vi "wrapper.vi"(8 "error in (no error)":errorcluster, 10 "Actor in":refnum<class "Actor.lvclass">, 11 "Change Frequency MSG in":refnum<class "Change Frequency MSG.lvclass">) -> (0 "error out":errorcluster, 3 "Actor out":refnum<class "Actor.lvclass">)   [LabVIEW 2014, in "Calibration.lvlib" / "Change Frequency MSG.lvclass"]
uses:
  Change Frequency MSG.lvclass
  <vilib>/ActorFramework/Actor/Actor.lvclass
  O3 Frequency Train Actor.lvclass
  SuperActor/SuperActor.lvclass/SuperActor.ctl
  O3 Frequency Train Actor.lvclass/O3 Frequency Train Actor.ctl
  Change Frequency MSG.lvclass/Change Frequency MSG.ctl
  SuperActor/Read CVT Session.vi
  SuperActor/Read Log Session.vi
  Accessors/Read FreqNotifier.vi
  <userlib>/_Session Fwk/Session - Root.lvclass
  reusable/Session APIs/Session Log/System Log.lvclass
  reusable/Session APIs/CVT/CVT.lvclass
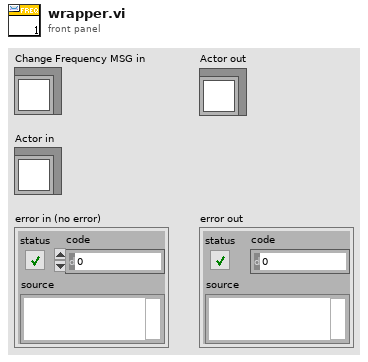
[diagram p1: front panel]
types:
  T1 = typedef "Session - Root.lvclass/Session Handle.ctl" = refnum<data-value>
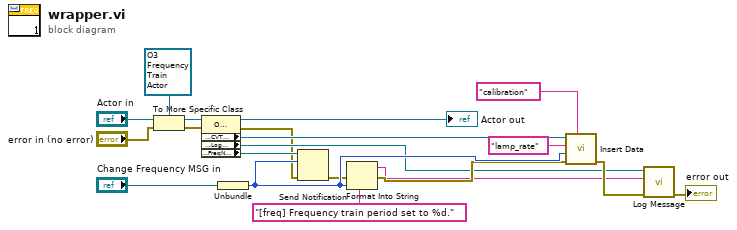
[diagram p0: block diagram]
diagram:
  n1 = To More Specific Class(target class=refnum<class "O3 Frequency Train Actor.lvclass"> refnum ("Calibration.lvlib:O3 Frequency Train Actors"), reference="Actor in", error in="error in (no error)") -> (specific class reference=w4:refnum<class "O3 Frequency Train Actor.lvclass">, error out=w5:errorcluster)
  n2 = property class="O3 Frequency Train Actors"(reference=w4, error in=w5) -> (reference out=→"Actor out":refnum<class "O3 Frequency Train Actor.lvclass">, error out=w7:errorcluster, "Accessors:CVT Session"=w15:T1, "Accessors:Log Session"=w14:T1, "Accessors:FreqNotifier"=w11:refnum<notifier>)
  n3 = Unbundle("Change Frequency MSG in") -> (w20:i64)
  n4 = Send Notification(notification=w20, notifier=w11, error in (no error)=w7) -> (error out=w13:errorcluster)  [unwired: 1 out]
  n5 = Format Into String(format string="[freq] Frequency train period set to %d.", error in=w13, w20) -> (resulting string=w9:string, error out=w16:errorcluster)  [unwired: 1 in]
  n6 = call "Insert Data.vi"("Group"="calibration", "error in"=w16, "Data"=w20, "tag"="lamp_rate", "CVT Session In"=w15) -> ("error out"=w17:errorcluster)  [unwired: 5 in, 1 out]
  n7 = call "Log Message.vi"("error in"=w17, "MSG In"=w9, "session in"=w14) -> ("error out"=→"error out":errorcluster)  [unwired: 7 in, 1 out]
